vi "IdentifyDIOChange.vi"(9 "Ctl Refnum":refnum<vi>, 10 "DIO Channel Array New":T1, 11 "DIO Channel Array Old":T1) -> (3 "Changed DIO":tag[](array[tag]))   [LabVIEW 2013]
uses:
  Controls/DIOChannels.ctl
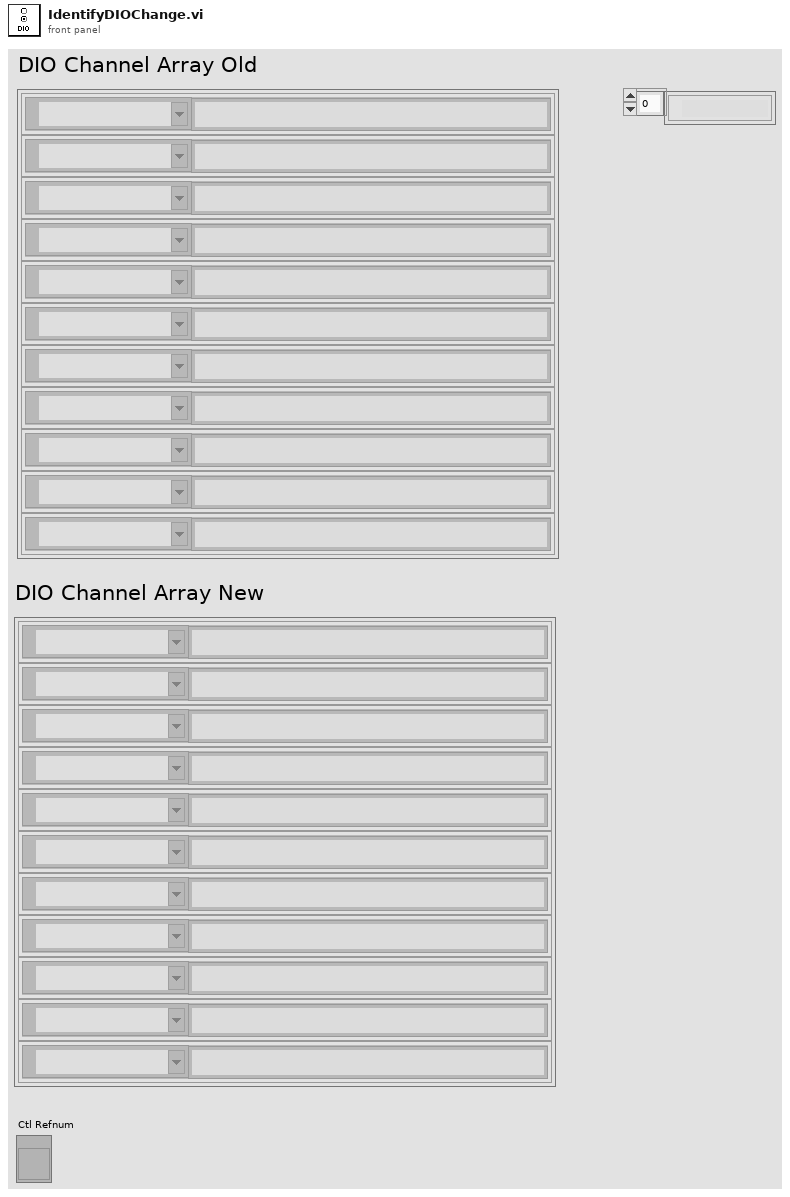
[diagram p1: front panel]
types:
  T1 = typedef "DIOChannels.ctl" = cluster{"Channel Name":string, "DIO lines":tag}[]
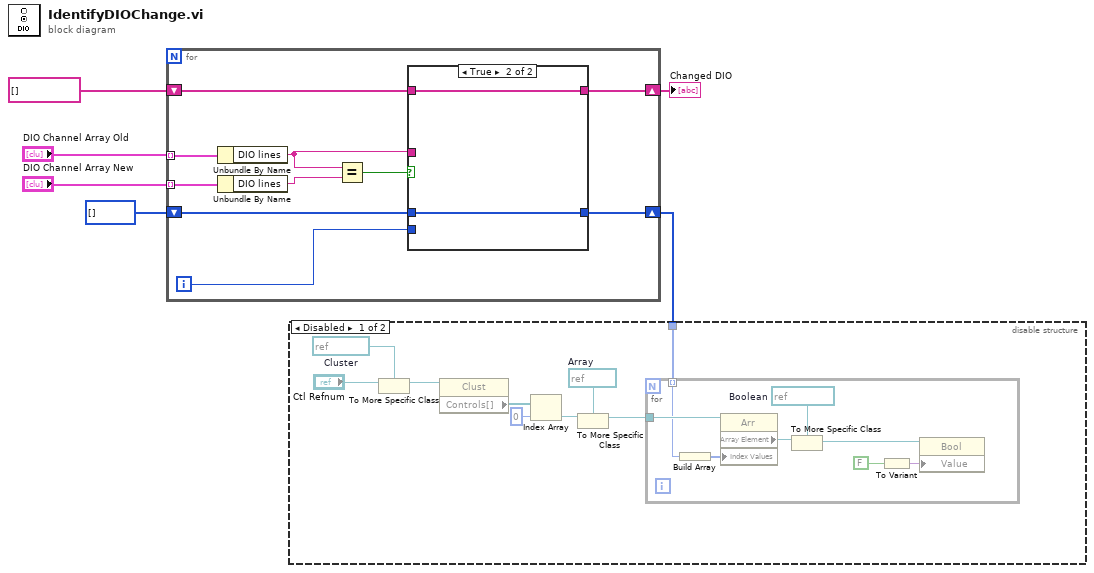
[diagram p0: block diagram]
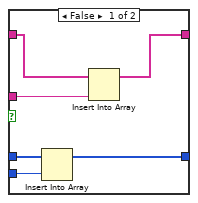
[diagram p3: hidden frame]
diagram:
  n1 = for {
    tunnel: "DIO Channel Array Old" -> [w16] mode=indexing
    tunnel: "DIO Channel Array New" -> [w15] mode=indexing
    shift-right: [w11] -> w6
    shift-left: tag[] [] -> [w10]
    shift-right: [w7] -> w1
    shift-left: i32[] [] -> [w8]
    i -> [w9]
    n2 = Unbundle By Name(w16) -> ("DIO lines"=w12:tag)
    n3 = Unbundle By Name(w15) -> ("DIO lines"=w14:tag)
    n4 = Equal?(x=w12, y=w14) -> (x = y?=w13:bool)
    n5 = case shown="True" w13 {
      tunnel: w12 -> [w22 _]
      tunnel: [w20 w24] -> w11
      tunnel: w10 -> [w21 w24]
      tunnel: w8 -> [w19 w23]
      tunnel: w9 -> [w18 _]
      tunnel: [w17 w23] -> w7
      frame False {
        n6 = Insert Into Array(array=w19, new element=w18) -> (w17:i32[])  [unwired: 1 in]
        n7 = Insert Into Array(array=w21, new element=w22) -> (w20:tag[])  [unwired: 1 in]
      }
      frame True {
      }
    }
  }
  "Changed DIO" <- w6
  n8 = disable-structure shown="Disabled" {
    disable-tunnel: w1 -> [w25 _]
    frame Disabled {
      w27 = refnum<vi> refnum  # Array
      w32 = refnum<vi> refnum  # Cluster
      n9 = To More Specific Class(target class=w32, reference="Ctl Refnum") -> (specific class reference=w31:refnum<vi>)  [unwired: 1 in, 1 out]
      n10 = property class="Clust"(reference=w31) -> ("Controls[]"=w30:refnum<vi>[])  [unwired: 1 in, 2 out]
      n11 = Index Array(array=w30, index=0) -> (element=w28:refnum<vi>)
      n12 = To More Specific Class(target class=w27, reference=w28) -> (specific class reference=w26:refnum<vi>)  [unwired: 1 in, 1 out]
      n13 = for {
        tunnel: w26 -> [w41]
        tunnel: w25 -> [w39] mode=indexing
        w37 = refnum<vi> refnum  # Boolean
        n14 = Build Array(w39) -> (w40:i32[])
        n15 = property class="Arr"(reference=w41, "Index Values"=w40) -> ("Array Element"=w38:refnum<vi>)  [unwired: 1 in, 2 out]
        n16 = To More Specific Class(target class=w37, reference=w38) -> (specific class reference=w36:refnum<vi>)  [unwired: 1 in, 1 out]
        n17 = To Variant(anything=FALSE) -> (Variant=w35:variant)
        n18 = property class="Bool"(reference=w36, "Value"=w35) -> ()  [unwired: 1 in, 2 out]
      }
    }
    frame Enabled {
    }
  }
